vi "DriverStationReadNumber.vi"(11 "Name":string="Numeric") -> (3 "output string":string)   [LabVIEW 2015]
uses:
  <vilib>/Rock Robotics/Network Tables/SD Read Number.vi
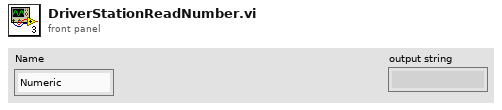
[diagram p1: front panel]
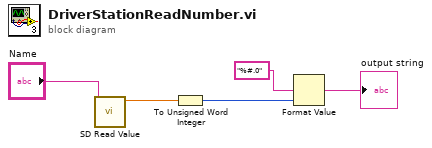
[diagram p0: block diagram]
diagram:
  n1 = call-poly <vilib>:"SD Read Value.vi"("Name"="Name") -> ("Numeric"=w4:dbl)  [unwired: 8 in, 2 out]
  n2 = To Unsigned Word Integer(number=w4) -> (unsigned 16bit integer=w3:u16)
  n3 = Format Value(format string="%#.0", value (0)=w3) -> (output string=→"output string":string)  [unwired: 1 in]
